vi "CMOS_DM_zernike-focalShift.vi"() -> ()   [LabVIEW 2020]
uses:
  C:/Users/Public/Documents/Photometrics/TPM-LabVIEWSamples/Examples/2020/Dependencies/PVCamNET.dll
  Dependencies/PVCamNET.dll
  <vilib>/numeric/Random Number (Range) U64.vi
  <vilib>/numeric/sub_Random U32.vi
  <vilib>/Utility/file.llb/Write Delimited Spreadsheet (DBL).vi
panel:
  in  "stop focal shift":bool
  out "Z_focalshift":dbl[](array[numeric])
  in  "Focal Shift1":dbl
  out "Focal Shift0":dbl
  in  "?":bool
  out "std":dbl[](array[numeric])
  out "Mirror":dbl[](array[numeric])
  out "Z_DM":dbl[](array[numeric])
  in  "stop iter":bool
  in  "pause iteration":bool
  in  "?":bool
  in  "?":bool
  in  "?":bool
  in  "?":bool
  out "Boolean":bool
  in  "error in":errorcluster
  out "Iter":i32
  out "Height":u16
  out "Width":u16
  out "Max":dbl
  out "Min":dbl
  in  "Exposure time":dbl=30.0
  in  "b2":dbl=5.0
  in  "b1":dbl=0.001
  in  "N":i32=1000
  in  "Path":path=path "C:/Users/Schererlab/Documents/Data/DZGong"
  out "XY Graph 2":cluster{i32[], dbl[]}(graph)
  out "error out":errorcluster
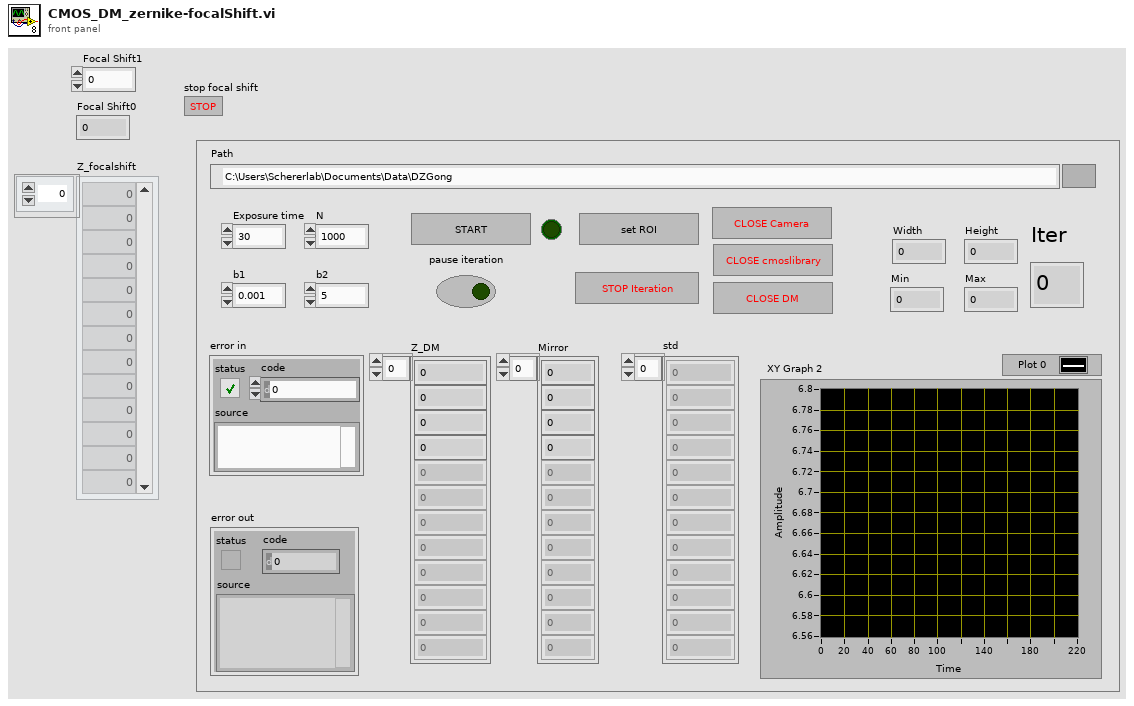
[diagram p1: front panel]
diagram:
  n1 = flat-sequence {
    tunnel: [w75] -> w65
    tunnel: [w74] -> w64
    tunnel: [w70] -> w40
    tunnel: [w69] -> w32
    tunnel: w65 -> [w83]
    tunnel: [w83] -> w63
    tunnel: w64 -> [w82]
    tunnel: [w82] -> w62
    tunnel: [w81] -> w41
    tunnel: w40 -> [w81]
    tunnel: [w80] -> w33
    tunnel: w32 -> [w80]
    tunnel: [w96] -> w61
    tunnel: [w97] -> w60
    tunnel: w63 -> [w97]
    tunnel: w62 -> [w96]
    tunnel: [w95] -> w42
    tunnel: w41 -> [w95]
    tunnel: [w94] -> w34
    tunnel: w33 -> [w94]
    tunnel: w61 -> [w103]
    tunnel: [w102] -> w59
    tunnel: w60 -> [w105]
    tunnel: [w104] -> w58
    tunnel: [w101] -> w43
    tunnel: w42 -> [w101]
    tunnel: [w100] -> w35
    tunnel: w34 -> [w100]
    tunnel: w59 -> [w109]
    tunnel: [w109] -> w57
    tunnel: w58 -> [w108]
    tunnel: [w108] -> w56
    tunnel: [w107] -> w44
    tunnel: w43 -> [w107]
    tunnel: [w106] -> w36
    tunnel: w35 -> [w106]
    tunnel: w57 -> [w117]
    tunnel: [w116] -> w55
    tunnel: w56 -> [w118]
    tunnel: [w118] -> w54
    tunnel: [w113] -> w45
    tunnel: w44 -> [w113]
    tunnel: [w112] -> w37
    tunnel: w36 -> [w112]
    tunnel: w55 -> [w124]
    tunnel: [w123] -> w53
    tunnel: w54 -> [w125]
    tunnel: [w125] -> w52
    tunnel: [w122] -> w46
    tunnel: w45 -> [w122]
    tunnel: [w121] -> w38
    tunnel: w37 -> [w121]
    tunnel: [w119] -> w27
    tunnel: w53 -> [w131]
    tunnel: [w131] -> w51
    tunnel: w52 -> [w130]
    tunnel: [w130] -> w50
    tunnel: [w128] -> w47
    tunnel: w46 -> [w128]
    tunnel: [w127] -> w39
    tunnel: w38 -> [w127]
    tunnel: w27 -> [w126]
    tunnel: [w126] -> w26
    tunnel: w51 -> [w144]
    tunnel: w50 -> [w142]
    tunnel: [w142] -> w23
    tunnel: [w143] -> w25
    tunnel: w47 -> [w140]
    tunnel: w39 -> [w139]
    tunnel: [w138] -> w21
    tunnel: [w137] -> w19
    tunnel: w26 -> [w135]
    tunnel: [w132] -> w17
    tunnel: w25 -> [w400]
    tunnel: [w400] -> w24
    tunnel: w23 -> [w399]
    tunnel: [w399] -> w22
    tunnel: w21 -> [w398]
    tunnel: [w398] -> w20
    tunnel: w19 -> [w397]
    tunnel: [w397] -> w18
    tunnel: w17 -> [w396]
    tunnel: w24 -> [w404]
    tunnel: [w404] -> w49
    tunnel: w22 -> [w403]
    tunnel: [w403] -> w48
    tunnel: w20 -> [w402]
    tunnel: [w402] -> w31
    tunnel: [w401] -> w30
    tunnel: w18 -> [w401]
    tunnel: w49 -> [w408]
    tunnel: w48 -> [w407]
    tunnel: w31 -> [w410]
    tunnel: w30 -> [w411]
    tunnel: [w411] -> w6
    tunnel: [w410] -> w4
    tunnel: [w407] -> w2
    tunnel: w6 -> [w415]
    tunnel: [w415] -> w5
    tunnel: w4 -> [w414]
    tunnel: [w414] -> w3
    tunnel: w2 -> [w413]
    tunnel: [w413] -> w1
    tunnel: w5 -> [w418]
    tunnel: [w416] -> w9
    tunnel: w3 -> [w419]
    tunnel: [w417] -> w8
    tunnel: w1 -> [w420]
    tunnel: [w420] -> w7
    tunnel: w9 -> [w456]
    tunnel: [w456] -> w16
    tunnel: w8 -> [w455]
    tunnel: [w455] -> w15
    tunnel: w7 -> [w454]
    tunnel: [w454] -> w10
    tunnel: w16 -> [w462]
    tunnel: [w462] -> w14
    tunnel: w15 -> [w461]
    tunnel: [w461] -> w12
    tunnel: w10 -> [w459]
    tunnel: w14 -> [w464]
    tunnel: [w464] -> w13
    tunnel: w12 -> [w463]
    tunnel: [w463] -> w11
    tunnel: w13 -> [w466]
    tunnel: [w466] -> w29
    tunnel: w11 -> [w465]
    tunnel: [w465] -> w28
    tunnel: w29 -> [w472]
    tunnel: w28 -> [w471]
    frame #0 {
      w72 = 0.0 ("Max")
      n2 = disable-structure shown="Disabled" {
        frame Disabled {
          n3 = call "SLM_init.vi"("dimension size y"=600 ("dimension size"), "dimension size x"=600 ("dimension size"), "Coordinates (screen)"=cluster{"X Position":i32, "Y Position":i32} {"X Position"=-700, "Y Position"=0}, "Window Number"=u8 0) -> ()  [unwired: 5 in, 1 out]
        }
        frame Enabled {
        }
      }
      n4 = call "DM_init.vi"("Error In"="error in") -> ("error out"=w69:errorcluster, "Mirror"=→"Mirror":dbl[], "instrument handle out"=w70:refnum<visa-resource-name>)  [unwired: 8 in]
      n5 = call "sCMOS_SingleAcq_init.vi"("Exposure time"="Exposure time") -> ("camera reference"=w74:refnum<k24>, "library reference"=w75:refnum<k24>)  [unwired: 9 in]
      "Boolean" <- FALSE ("Boolean")
      "Max" <- w72
      "Min" <- w72
      "Z_DM" <- dbl[] [0.0, 0.0, 0.0, 0.0, 0.0, 0.0, 0.0, 0.0, 0.0, 0.0, 0.0, 0.0, 0.0, 0.0, 0.0] ("Coefficient")
    }
    frame #1 {
      n6 = disable-structure shown="Disabled" {
        frame Disabled {
          n7 = for {
            N: 60 -> [_]
            tunnel: [w89] -> w84 mode=indexing
            n8 = for {
              N: 60 -> [_]
              tunnel: [w91] -> w89 mode=indexing
              n9 = call-poly <vilib>:"Random Number (Range).vi"("lower bound (0)"=u64 0, "upper bound (100)"=u64 255) -> ("number"=w91:u64)  [unwired: 9 in]
            }
          }
          n10 = call "RandomMask_gen.vi"("scale factor"=10, "X"=w84) -> ("Y"=w86:dbl[][])  [unwired: 9 in]
          n11 = call "SLM_display.vi"("mask"=w86, "Window Number"=u8 0) -> ()  [unwired: 10 in]
        }
        frame Enabled {
        }
      }
    }
    frame #2 {
      n12 = while {
        stop <- "?" stop-if-true
        n13 = Wait (ms)(milliseconds to wait=u32 100) -> ()  [unwired: 1 out]
        n14 = local write "Boolean"("?") -> ()
      }
    }
    frame #3 {
      n15 = call "sCMOS_SingleAcq_ShowImage.vi"("camera refernce"=w103, "library reference in"=w105) -> ("library reference out"=w104:refnum<k24>)  [unwired: 9 in]
      n16 = call "sCMOS_SingleAcq_AcqImage.vi"("camera reference in"=w103) -> ("camerareference out"=w102:refnum<k24>)  [unwired: 7 in, 3 out]
    }
    frame #4 {
      n17 = while {
        stop <- "?" stop-if-true
        n18 = Wait (ms)(milliseconds to wait=u32 100) -> ()  [unwired: 1 out]
      }
    }
    frame #5 {
      n19 = call "sCMOS_SingleAcq_ROI.vi"("camera reference input"=w117) -> ("Width"=→"Width":u16, "Height"=→"Height":u16, "camera reference output"=w116:refnum<k24>)  [unwired: 6 in]
    }
    frame #6 {
      n20 = call "sCMOS_SingleAcq_AcqImage.vi"("camera reference in"=w124) -> ("RawImageData"=w120:u16[], "camerareference out"=w123:refnum<k24>)  [unwired: 7 in, 2 out]
      n21 = call "STD.vi"("Array"=w120) -> ("Numeric"=w119:dbl)
    }
    frame #7 {
      n22 = Wait (ms)(milliseconds to wait=u32 200) -> ()  [unwired: 1 out]
    }
    frame #8 {
      n23 = Initialize Array(w135, 1 ("dimension size")) -> (w134:dbl[])
      n24 = for {
        N: "N" -> [_]
        tunnel: w144 -> [w225]
        tunnel: [w217] -> w143
        tunnel: w140 -> [w215]
        tunnel: w139 -> [w212]
        tunnel: [w209] -> w138
        tunnel: [w208] -> w137
        shift-right: [w199] -> _
        shift-left: w134 -> [w202]
        shift-right: [w200] -> _
        shift-left: i32[] [] -> [w201]
        tunnel: [w176] -> w132 mode=indexing
        i -> [w175]
        stop <- w207 stop-if-true
        n25 = flat-sequence {
          tunnel: [w228] -> w222
          tunnel: [w227] -> w221
          tunnel: w225 -> [w228]
          tunnel: w222 -> [w248]
          tunnel: [w248] -> w152
          tunnel: w221 -> [w244]
          tunnel: [w244] -> w150
          tunnel: w215 -> [w241]
          tunnel: [w240] -> w148
          tunnel: w212 -> [w239]
          tunnel: [w238] -> w146
          tunnel: w152 -> [w253]
          tunnel: [w253] -> w151
          tunnel: w150 -> [w252]
          tunnel: [w252] -> w149
          tunnel: w148 -> [w251]
          tunnel: [w251] -> w147
          tunnel: w146 -> [w250]
          tunnel: [w250] -> w145
          tunnel: w151 -> [w255]
          tunnel: [w254] -> w156
          tunnel: w149 -> [w258]
          tunnel: [w258] -> w155
          tunnel: w147 -> [w257]
          tunnel: [w257] -> w154
          tunnel: w145 -> [w256]
          tunnel: [w256] -> w153
          tunnel: w156 -> [w263]
          tunnel: [w263] -> w224
          tunnel: w155 -> [w262]
          tunnel: [w262] -> w223
          tunnel: [w261] -> w213
          tunnel: w154 -> [w261]
          tunnel: [w260] -> w211
          tunnel: w153 -> [w260]
          tunnel: w224 -> [w270]
          tunnel: w223 -> [w269]
          tunnel: [w269] -> w198
          tunnel: [w266] -> w196
          tunnel: [w268] -> w194
          tunnel: [w265] -> w192
          tunnel: w213 -> [w265]
          tunnel: [w264] -> w190
          tunnel: w211 -> [w264]
          tunnel: w198 -> [w276]
          tunnel: [w276] -> w197
          tunnel: w196 -> [w275]
          tunnel: [w275] -> w195
          tunnel: w194 -> [w274]
          tunnel: [w274] -> w193
          tunnel: w192 -> [w273]
          tunnel: [w273] -> w191
          tunnel: w190 -> [w272]
          tunnel: [w272] -> w189
          tunnel: w197 -> [w284]
          tunnel: [w284] -> w166
          tunnel: w195 -> [w288]
          tunnel: [w288] -> w164
          tunnel: [w283] -> w162
          tunnel: w193 -> [w283]
          tunnel: [w280] -> w160
          tunnel: w191 -> [w279]
          tunnel: w189 -> [w278]
          tunnel: [w277] -> w158
          tunnel: w166 -> [w294]
          tunnel: [w294] -> w165
          tunnel: w164 -> [w293]
          tunnel: [w293] -> w163
          tunnel: w162 -> [w292]
          tunnel: [w292] -> w161
          tunnel: w160 -> [w291]
          tunnel: [w291] -> w159
          tunnel: w158 -> [w290]
          tunnel: [w290] -> w157
          tunnel: w165 -> [w300]
          tunnel: [w300] -> w171
          tunnel: w163 -> [w299]
          tunnel: [w299] -> w170
          tunnel: w161 -> [w296]
          tunnel: [w295] -> w169
          tunnel: w159 -> [w298]
          tunnel: [w298] -> w168
          tunnel: w157 -> [w297]
          tunnel: [w297] -> w167
          tunnel: w171 -> [w306]
          tunnel: [w306] -> w220
          tunnel: w170 -> [w305]
          tunnel: [w305] -> w219
          tunnel: [w304] -> w218
          tunnel: w169 -> [w304]
          tunnel: w168 -> [w303]
          tunnel: [w303] -> w214
          tunnel: [w302] -> w210
          tunnel: w167 -> [w302]
          tunnel: w220 -> [w314]
          tunnel: [w314] -> w188
          tunnel: w219 -> [w313]
          tunnel: [w313] -> w186
          tunnel: w218 -> [w312]
          tunnel: [w311] -> w184
          tunnel: [w309] -> w182
          tunnel: w214 -> [w308]
          tunnel: [w308] -> w180
          tunnel: [w307] -> w178
          tunnel: w210 -> [w307]
          tunnel: w188 -> [w321]
          tunnel: [w321] -> w187
          tunnel: w186 -> [w320]
          tunnel: [w320] -> w185
          tunnel: w184 -> [w319]
          tunnel: [w319] -> w183
          tunnel: w182 -> [w318]
          tunnel: [w318] -> w181
          tunnel: w180 -> [w317]
          tunnel: [w317] -> w179
          tunnel: w178 -> [w316]
          tunnel: [w316] -> w177
          tunnel: w187 -> [w333]
          tunnel: w185 -> [w330]
          tunnel: [w332] -> w173
          tunnel: w183 -> [w332]
          tunnel: w181 -> [w329]
          tunnel: [w328] -> _
          tunnel: w179 -> [w325]
          tunnel: w177 -> [w324]
          tunnel: [w323] -> w209
          tunnel: [w322] -> w208
          tunnel: w201 -> [_]
          tunnel: w173 -> [w342]
          tunnel: [w342] -> w172
          tunnel: w172 -> [w344]
          tunnel: [w343] -> w174
          tunnel: w174 -> [w345]
          tunnel: [w345] -> w216
          tunnel: w216 -> [w360]
          tunnel: w175 -> [w358]
          tunnel: [w359] -> w206
          tunnel: [w351] -> w204
          tunnel: w175 -> [w348]
          tunnel: w206 -> [w378]
          tunnel: [w378] -> w205
          tunnel: w204 -> [w372]
          tunnel: [w372] -> w203
          tunnel: w202 -> [w377]
          tunnel: w201 -> [w376]
          tunnel: w175 -> [w374]
          tunnel: [w363] -> w200
          tunnel: [w370] -> w199
          tunnel: [w381] -> w217
          tunnel: w205 -> [w381]
          tunnel: w203 -> [w379]
          tunnel: [w380] -> w207
          tunnel: [w379] -> w176
          frame #0 {
            n26 = for {
              N: 12 -> [_]
              tunnel: [w232] -> w227 mode=indexing
              n27 = call-poly <vilib>:"Random Number (Range).vi"("lower bound (0)"=u64 0, "upper bound (100)"=u64 1) -> ("number"=w237:u64)  [unwired: 9 in]
              n28 = Subtract(x=w237, y=0.5) -> (x-y=w235:dbl)
              n29 = Multiply(x=w235, y=2.0) -> (x*y=w233:dbl)
              n30 = Multiply(x=w233, y="b1") -> (x*y=w232:dbl)
            }
          }
          frame #1 {
            n31 = local read "Z_DM"() -> (w247:dbl[])
            n32 = Add(x=w244, y=w247) -> (x+y=w243:dbl[])
            n33 = call "range_filter.vi"("array input"=w243, "upper limit"=1.0, "lower limit"=-1.0) -> ("Array output"=w242:dbl[])  [unwired: 7 in]
            n34 = call "DM_excute.vi"("error in (no error)"=w239, "Zernike Amplitudes"=w242, "instrument handle"=w241) -> ("error out"=w238:errorcluster, "instrument handle out"=w240:refnum<visa-resource-name>)  [unwired: 5 in, 2 out]
          }
          frame #2 {
            n35 = Wait (ms)(milliseconds to wait=u32 100) -> ()  [unwired: 1 out]
          }
          frame #3 {
            n36 = call "sCMOS_SingleAcq_AcqImage.vi"("camera reference in"=w255) -> ("camerareference out"=w254:refnum<k24>)  [unwired: 7 in, 3 out]
          }
          frame #4 {
            n37 = Wait (ms)(milliseconds to wait=u32 100) -> ()  [unwired: 1 out]
          }
          frame #5 {
            n38 = call "sCMOS_SingleAcq_AcqImage.vi"("camera reference in"=w270) -> ("RawImageData"=w267:u16[], "camerareference out"=w268:refnum<k24>)  [unwired: 7 in, 2 out]
            n39 = call "STD.vi"("Array"=w267) -> ("Numeric"=w266:dbl)
          }
          frame #6 {
            n40 = Wait (ms)(milliseconds to wait=u32 100) -> ()  [unwired: 1 out]
          }
          frame #7 {
            n41 = local read "Z_DM"() -> (w285:dbl[])
            n42 = Subtract(x=w285, y=w284) -> (x-y=w282:dbl[])
            n43 = call "range_filter.vi"("array input"=w282, "upper limit"=1.0, "lower limit"=-1.0) -> ("Array output"=w281:dbl[])  [unwired: 7 in]
            n44 = call "DM_excute.vi"("error in (no error)"=w278, "Zernike Amplitudes"=w281, "instrument handle"=w279) -> ("error out"=w277:errorcluster, "instrument handle out"=w280:refnum<visa-resource-name>)  [unwired: 5 in, 2 out]
          }
          frame #8 {
            n45 = Wait (ms)(milliseconds to wait=u32 100) -> ()  [unwired: 1 out]
          }
          frame #9 {
            n46 = call "sCMOS_SingleAcq_AcqImage.vi"("camera reference in"=w296) -> ("camerareference out"=w295:refnum<k24>)  [unwired: 7 in, 3 out]
          }
          frame #10 {
            n47 = Wait (ms)(milliseconds to wait=u32 100) -> ()  [unwired: 1 out]
          }
          frame #11 {
            n48 = call "sCMOS_SingleAcq_AcqImage.vi"("camera reference in"=w312) -> ("RawImageData"=w310:u16[], "camerareference out"=w311:refnum<k24>)  [unwired: 7 in, 2 out]
            n49 = call "STD.vi"("Array"=w310) -> ("Numeric"=w309:dbl)
          }
          frame #12 {
            n50 = Wait (ms)(milliseconds to wait=u32 100) -> ()  [unwired: 1 out]
          }
          frame #13 {
            n51 = Subtract(x=w330, y=w329) -> (x-y=w336:dbl)
            n52 = Greater?(x=w330, y=w329) -> (0:w331:bool)
            n53 = Multiply(x=w336, y=w333) -> (x*y=w337:dbl[])
            n54 = Select(t=w330, s=w331, f=w329) -> (s? t:f=w328:dbl)
            n55 = Multiply(x=w337, y="b2") -> (x*y=w338:dbl[])
            n56 = local read "Z_DM"() -> (w340:dbl[])
            n57 = Add(x=w340, y=w338) -> (x+y=w327:dbl[])
            n58 = call "range_filter.vi"("array input"=w327, "upper limit"=1.0, "lower limit"=-1.0) -> ("Array output"=w326:dbl[])  [unwired: 7 in]
            n59 = local write "Z_DM"(w326) -> ()
            n60 = call "DM_excute.vi"("error in (no error)"=w324, "Zernike Amplitudes"=w326, "instrument handle"=w325) -> ("error out"=w322:errorcluster, "instrument handle out"=w323:refnum<visa-resource-name>)  [unwired: 5 in, 2 out]
          }
          frame #14 {
            n61 = Wait (ms)(milliseconds to wait=u32 100) -> ()  [unwired: 1 out]
          }
          frame #15 {
            n62 = call "sCMOS_SingleAcq_AcqImage.vi"("camera reference in"=w344) -> ("camerareference out"=w343:refnum<k24>)  [unwired: 7 in, 3 out]
          }
          frame #16 {
          }
          frame #17 {
            n63 = call "sCMOS_SingleAcq_AcqImage.vi"("camera reference in"=w360) -> ("RawImageData"=w349:u16[], "camerareference out"=w359:refnum<k24>)  [unwired: 7 in, 2 out]
            n64 = Path To String(path="Path") -> (string=w346:string)
            n65 = local read "Height"() -> (w362:u16)
            n66 = local read "Width"() -> (w361:u16)
            n67 = Number To Decimal String(number=w358) -> (decimal integer string=w357:string)  [unwired: 1 in]
            n68 = Array Max & Min(array=w349) -> (max value=w354:u16)  [unwired: 3 out]
            n69 = Reshape Array(w349, w362, w361) -> (w350:u16[][])
            n70 = Concatenate Strings(w346, "\\DM_zernike_", w357, ".png" ("string")) -> (w355:string)
            n71 = Divide(x=w350, y=w354) -> (x/y=w353:dbl[][])
            n72 = call "STD.vi"("Array"=w349) -> ("Numeric"=w351:dbl)
            n73 = call "MatLab_imwrite.vi"("image"=w353, "path"=w355) -> ()  [unwired: 10 in]
            "Iter" <- w348
          }
          frame #18 {
            n74 = Add(x=1, y=w374) -> (x+y=w373:i32)
            n75 = Build Array (concatenate)(w376, w373) -> (w363:i32[])
            n76 = Build Array (concatenate)(w377, w372) -> (w370:dbl[])
            n77 = Delete From Array(array=w370, length=1, index=0) -> (array with subset deleted=w364:dbl[])  [unwired: 1 out]
            n78 = Delete From Array(array=w363, length=1, index=0) -> (array with subset deleted=w365:i32[])  [unwired: 1 out]
            n79 = Bundle(w365, w364) -> (→"XY Graph 2":cluster{i32[], dbl[]})  [unwired: 1 in]
          }
          frame #19 {
            n80 = while {
              tunnel: ["stop iter"] -> w380
              stop <- w383 stop-if-true
              n81 = Wait (ms)(milliseconds to wait=u32 20) -> ()  [unwired: 1 out]
              n82 = Not(x="pause iteration") -> (.not. x?=w384:bool)
              n83 = Or(x=w384, y="stop iter") -> (x .or. y?=w383:bool)
            }
          }
        }
      }
      "std" <- w132
    }
    frame #9 {
      n84 = local read "Path"() -> (w389:path)
      n85 = local read "Z_DM"() -> (w393:dbl[])
      n86 = Path To String(path=w389) -> (string=w391:string)
      n87 = Concatenate Strings(w391, "\\zernike.txt" ("string")) -> (w390:string)
      n88 = Concatenate Strings(w391, "\\std.txt" ("string")) -> (w394:string)
      n89 = String To Path(string=w390) -> (path=w387:path)
      n90 = call-poly <vilib>:"Write Delimited Spreadsheet.vi"("file path (dialog if empty)"=w387, "1D data"=w393) -> ()  [unwired: 12 in, 2 out]
      n91 = String To Path(string=w394) -> (path=w388:path)
      n92 = call-poly <vilib>:"Write Delimited Spreadsheet.vi"("file path (dialog if empty)"=w388, "1D data"=w396) -> ()  [unwired: 12 in, 2 out]
    }
    frame #10 {
      n93 = while {
        stop <- "?" stop-if-true
        n94 = Wait (ms)(milliseconds to wait=u32 100) -> ()  [unwired: 1 out]
      }
    }
    frame #11 {
      n95 = invoke class="Camera" method="Close"(reference=w408) -> (reference out=w409:refnum<k24>)  [unwired: 2 in, 2 out]
      n96 = Close Reference(reference=w409) -> ()  [unwired: 1 in, 1 out]
    }
    frame #12 {
      "Focal Shift0" <- 0.0 ("Focal Shift0")
    }
    frame #13 {
      n97 = while {
        tunnel: w419 -> [w425]
        tunnel: w418 -> [w424]
        tunnel: [w423] -> w417
        tunnel: [w422] -> w416
        stop <- w421 stop-if-true
        n98 = flat-sequence {
          tunnel: ["Focal Shift1"] -> w427
          tunnel: [w428] -> w426
          tunnel: w427 -> [w436]
          tunnel: w426 -> [w435]
          tunnel: w425 -> [w434]
          tunnel: w424 -> [w433]
          tunnel: [w432] -> w423
          tunnel: [w431] -> w422
          tunnel: ["stop focal shift"] -> w421
          frame #0 {
            n99 = local read "Focal Shift0"() -> (w429:dbl)
            n100 = Not Equal?(x="Focal Shift1", y=w429) -> (x != y?=w428:bool)
          }
          frame #1 {
            n101 = case shown="True" w435 {
              tunnel: w436 -> [_ w446]
              tunnel: w434 -> [w437 w443]
              tunnel: w433 -> [w438 w442]
              tunnel: [w437 w441] -> w432
              tunnel: [w438 w440] -> w431
              frame False {
              }
              frame True {
                n102 = local read "Z_DM"() -> (w450:dbl[])
                n103 = local write "Focal Shift0"(w446) -> ()
                n104 = Array Subset(array=w450, index=1, length=1) -> (w447:dbl[])
                n105 = Add(x=w447, y=w446) -> (x+y=w445:dbl[])
                n106 = Replace Array Subset(array=w450, new element=w445, index=1) -> (w444:dbl[])
                n107 = call "DM_excute.vi"("error in (no error)"=w442, "Zernike Amplitudes"=w444, "instrument handle"=w443) -> ("error out"=w440:errorcluster, "ZernikePattern"=→"Z_focalshift":dbl[], "instrument handle out"=w441:refnum<visa-resource-name>)  [unwired: 5 in, 1 out]
              }
            }
          }
          frame #2 {
            n108 = Wait (ms)(milliseconds to wait=u32 100) -> ()  [unwired: 1 out]
          }
        }
      }
    }
    frame #14 {
      n109 = while {
        stop <- "?" stop-if-true
        n110 = Wait (ms)(milliseconds to wait=u32 100) -> ()  [unwired: 1 out]
      }
    }
    frame #15 {
      n111 = invoke class="Library" method="Release"(reference=w459) -> (reference out=w460:refnum<k24>)  [unwired: 2 in, 2 out]
      n112 = Close Reference(reference=w460) -> ()  [unwired: 1 in, 1 out]
    }
    frame #16 {
      n113 = invoke class="GC" method="Collect"() -> ()  [unwired: 3 in, 3 out]
    }
    frame #17 {
      n114 = while {
        stop <- "?" stop-if-true
        n115 = Wait (ms)(milliseconds to wait=u32 100) -> ()  [unwired: 1 out]
      }
    }
    frame #18 {
      n116 = local write "Boolean"(FALSE ("Boolean")) -> ()
      n117 = call "DM_release.vi"("error in (no error)"=w472, "instrument handle"=w471) -> ("error out"=→"error out":errorcluster, "Mirror"=w469:dbl[])  [unwired: 8 in]
      n118 = disable-structure shown="Disabled" {
        frame Disabled {
          n119 = call "SLM_release.vi"("Window Number"=0) -> ()  [unwired: 11 in]
        }
        frame Enabled {
        }
      }
      n120 = local write "Mirror"(w469) -> ()
    }
  }
